vi "DAQ6363_RecordGraph.vi"() -> ()   [LabVIEW 2019]
panel:
  out "CHs Ratio":dbl
  out "Delta Counts":dbl
  in  "Clear":bool
  out "Data2":T1
  in  "Ch 2":enum16{"Ch1", "Ch2", "Ch3", "Ch4"}(ring)=enum."Ch2"
  in  "Max T(s)":i32=1 min=1 max=10000 step=1
  in  "Show Avg":bool
  in  "Avg Val":i32=1 min=1 max=10000 step=1
  in  "DataIn":T2(array[cluster])
  in  "Ch":enum16{"Ch1", "Ch2", "Ch3", "Ch4"}(ring)
  out "Data":T1
  in  "error in (no error)":errorcluster caption="entrée d'erreur (pas d'erreur)"
  out "Graph":T3(graph)
  out "error out":errorcluster caption="sortie d'erreur"
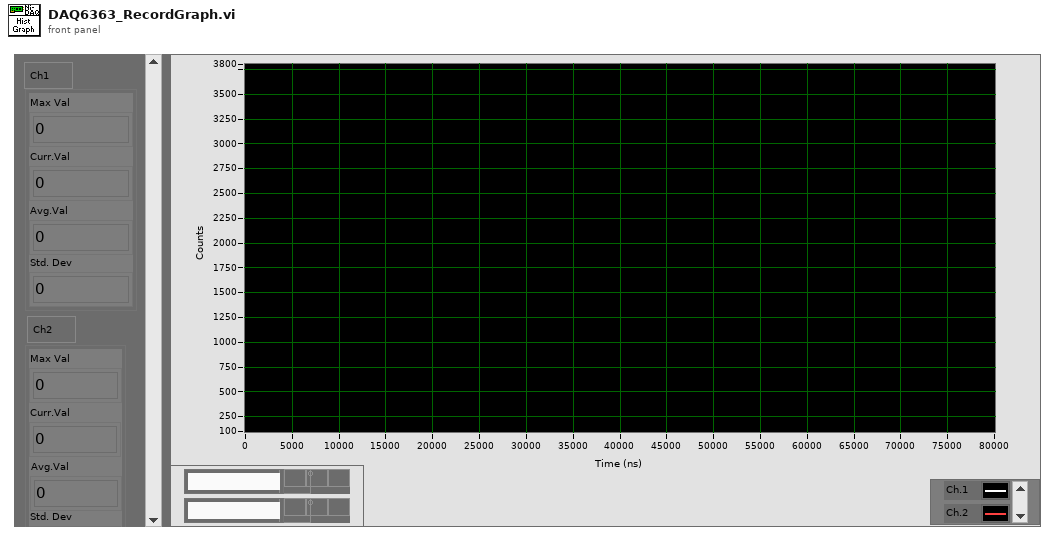
[diagram p1: front panel]
types:
  T1 = cluster{"Max Val":dbl, "Curr.Val":dbl, "Avg.Val":dbl, "Std. Dev":dbl}
  T2 = cluster{"Max Val":dbl, "Curr.Val":dbl, "Avg.Val":dbl, "Std. Dev":dbl}[]
  T3 = cluster{dbl, "Resolution (ns)":dbl, "Histogram":u32[][]}
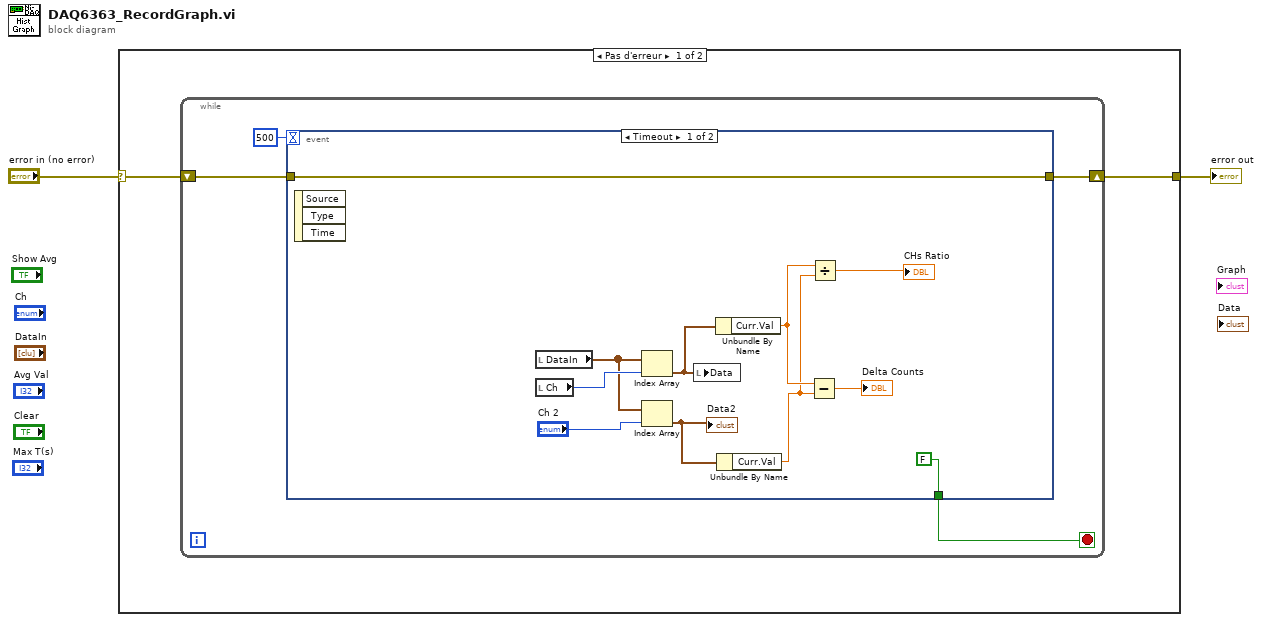
[diagram p0: block diagram]
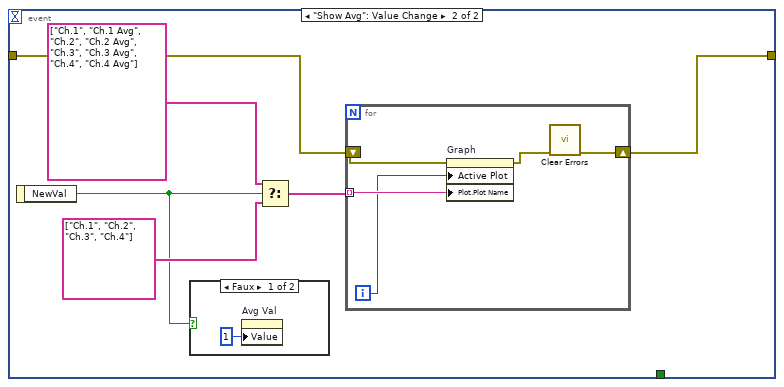
[diagram p2: hidden frame]
diagram:
  n1 = case shown="Pas d'erreur" "error in (no error)" {
    selector: "error in (no error)" -> [w3 w32]
    tunnel: [w4 w32] -> w2
    frame No Error {
      n2 = while {
        shift-right: [w7] -> w4
        shift-left: w3 -> [w6]
        stop <- w5 stop-if-true
        n3 = event shown="[0] Timeout" {
          selector: _ -> [_ _]
          dyn-events: _ -> [_ _]
          timeout: 500 -> [_ _]
          tunnel: [w19 w21] -> w7
          tunnel: w6 -> [w19 w22]
          tunnel: [FALSE _] -> w5
          event Timeout {
            n4 = event-data() -> ()  [unwired: 1 in, 3 out]
            n5 = local read "DataIn"() -> (w16:T2)
            n6 = local read "Ch"() -> (w17:enum16{"Ch1", "Ch2", "Ch3", "Ch4"})
            n7 = Index Array(array=w16, index=w17) -> (element=w14:T1)
            n8 = Index Array(array=w16, index="Ch 2") -> (element=w13:T1)
            "Data2" <- w13
            n9 = local write "Data"(w14) -> ()
            n10 = Unbundle By Name(w14) -> ("Curr.Val"=w11:dbl)
            n11 = Unbundle By Name(w13) -> ("Curr.Val"=w10:dbl)
            n12 = Subtract(x=w11, y=w10) -> (x-y=→"Delta Counts":dbl)
            n13 = Divide(x=w11, y=w10) -> (x/y=→"CHs Ratio":dbl)
          }
          event "Show Avg": Value Change {
            n14 = event-data() -> ("NewVal"=w20:bool)  [unwired: 1 in]
            n15 = case shown="Faux" w20 {
              frame False {
                n16 = property on="Avg Val" class="NumNb (strict)"("Value"=1 ("Avg Val")) -> ()  [unwired: 2 in, 2 out]
              }
              frame True {
              }
            }
            n17 = Select(t=string[] ["Ch.1", "Ch.1 Avg", "Ch.2", "Ch.2 Avg", "Ch.3", "Ch.3 Avg", "Ch.4", "Ch.4 Avg"], s=w20, f=string[] ["Ch.1", "Ch.2", "Ch.3", "Ch.4"]) -> (s? t:f=w23:string[])
            n18 = for {
              tunnel: w23 -> [w31] mode=indexing
              shift-right: [w28] -> w21
              shift-left: w22 -> [w30]
              i -> [w27]
              n19 = property on="Graph" class="GraphWF (strict)"(error in=w30, "Active Plot"=w27, "Plot.Plot Name"=w31) -> (error out=w29:errorcluster)  [unwired: 1 in, 1 out]
              n20 = call <vilib>:"Clear Errors.vi"("error in (no error)"=w29) -> ("error out"=w28:errorcluster)  [unwired: 5 in, 1 out]
            }
          }
        }
      }
    }
    frame Error {
    }
  }
  "error out" <- w2
